vi "test first time creates file.vi"(8 "error in (no error)":errorcluster, 11 "TestCase in":refnum<class "Testing Approval Tests.lvclass">) -> (0 "error out":errorcluster, 3 "TestCase out":refnum<class "Testing Approval Tests.lvclass">)   [LabVIEW 2020, in "Testing Approval Tests.lvclass"]
uses:
  Testing Approval Tests.lvclass
  <vilib>/addons/_JKI Toolkits/VI Tester/TestCase.llb/TestCase.lvclass
  C:/Program Files/National Instruments/LabVIEW 2020/vi.lib/addons/_JKI Toolkits/VI Tester/TestCase.llb/TestCase.lvclass
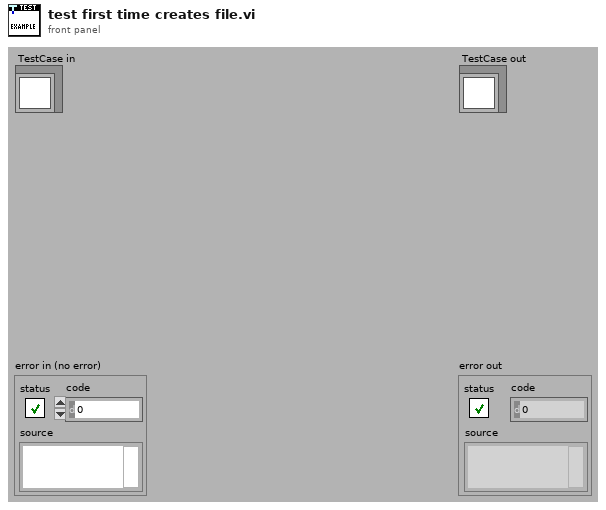
[diagram p1: front panel]
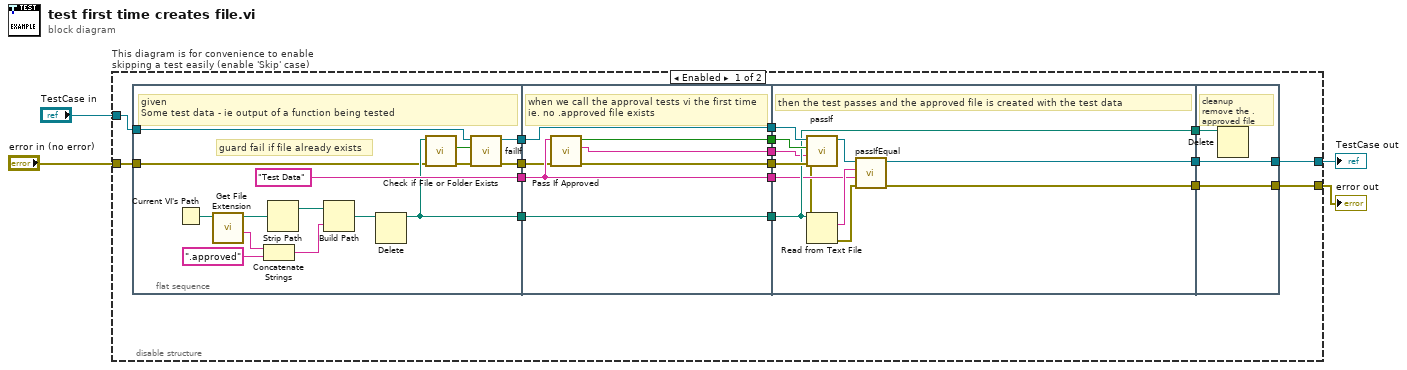
[diagram p0: block diagram]
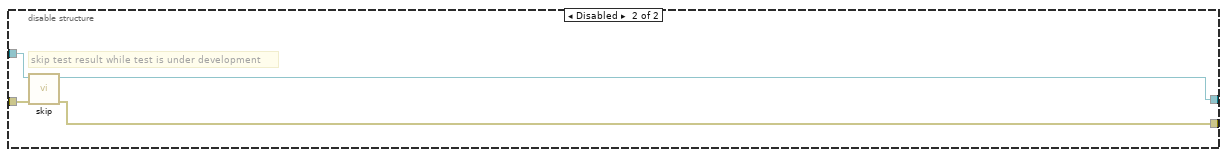
[diagram p2: hidden frame]
diagram:
  n1 = disable-structure "This diagram is for convenience to enable skipping a test easily (enable 'Skip' case)" shown="Enabled" {
    disable-tunnel: "TestCase in" -> [w19 w62]
    disable-tunnel: [w17 w60] -> w1
    disable-tunnel: [w13 w61] -> w3
    disable-tunnel: "error in (no error)" -> [w16 w59]
    frame Enabled {
      n2 = flat-sequence {
        tunnel: [w26] -> w20
        tunnel: w19 -> [w27]
        tunnel: w16 -> [w24]
        tunnel: [w28] -> w15
        tunnel: ["Test Data"] -> w10
        tunnel: [w25] -> w8
        tunnel: [w43] -> w21
        tunnel: w20 -> [w43]
        tunnel: w15 -> [w39]
        tunnel: [w38] -> w14
        tunnel: [w42] -> w11
        tunnel: w10 -> [w40]
        tunnel: [w41] -> w9
        tunnel: w8 -> [w41]
        tunnel: [w40] -> w6
        tunnel: [w37] -> w5
        tunnel: w21 -> [w55]
        tunnel: [w49] -> w18
        tunnel: w14 -> [w53]
        tunnel: [w51] -> w12
        tunnel: w11 -> [w54]
        tunnel: w9 -> [w52]
        tunnel: [w52] -> w7
        tunnel: w6 -> [w47]
        tunnel: w5 -> [w45]
        tunnel: w18 -> [w58]
        tunnel: [w58] -> w17
        tunnel: [w57] -> w13
        tunnel: w12 -> [w57]
        tunnel: w7 -> [w56]
        frame #0 {
          # "guard fail if file already exists"
          # "given\nSome test data - ie output of a function being tested"
          n3 = Current VI's Path() -> (path=w35:path)
          n4 = call <vilib>:"Get File Extension.vi"("file"=w35) -> ("filename without extension"=w32:string, "dup file"=w34:path)  [unwired: 6 in, 3 out]
          n5 = Concatenate Strings(w32, ".approved" ("string")) -> (w30:string)
          n6 = Strip Path(path=w34) -> (stripped path=w33:path)  [unwired: 1 out]
          n7 = Build Path(base path=w33, name or relative path=w30) -> (appended path=w29:path)
          n8 = Delete(path (use dialog)=w29) -> (deleted path=w25:path)  [unwired: 4 in, 2 out]
          n9 = call <vilib>:"Check if File or Folder Exists.vi"("error in (no error)"=w24, "path"=w25) -> ("error out"=w23:errorcluster, "file or folder exists?"=w22:bool)  [unwired: 7 in, 1 out]
          n10 = call-dynamic "failIf.vi"("error in (no error)"=w23, "fail"=w22, "TestCase in"=w27) -> ("error out"=w28:errorcluster, "TestCase out"=w26:refnum<class "Testing Approval Tests.lvclass">)  [unwired: 7 in]
        }
        frame #1 {
          # "when we call the approval tests vi the first time\nie. no .approved file exists"
          n11 = call "Pass If Approved.vi"("error in (no error)"=w39, "Test Data"=w40) -> ("error out"=w38:errorcluster, "Failure Message"=w37:string, "Passed?"=w42:bool)  [unwired: 7 in]
        }
        frame #2 {
          # "then the test passes and the approved file is created with the test data"
          n12 = call-dynamic "passIf.vi"("error in (no error)"=w53, "message (\"\")"=w45, "pass"=w54, "TestCase in"=w55) -> ("error out"=w44:errorcluster, "TestCase out"=w50:refnum<class "Testing Approval Tests.lvclass">)  [unwired: 6 in]
          n13 = Read from Text File(file (use dialog)=w52, error in=w44) -> (text=w48:string, error out=w46:errorcluster)  [unwired: 2 in, 2 out]
          n14 = call-dynamic "passIfEqual.vi"("error in (no error)"=w46, "y"=w47, "x"=w48, "TestCase in"=w50) -> ("error out"=w51:errorcluster, "TestCase out"=w49:refnum<class "Testing Approval Tests.lvclass">)  [unwired: 6 in]
        }
        frame #3 {
          # "cleanup \nremove the .approved file"
          n15 = Delete(path (use dialog)=w56) -> ()  [unwired: 4 in, 3 out]
        }
      }
    }
    frame Disabled {
      # "skip test result while test is under development"
      n16 = call <vilib>:"skip.vi"("error in (no error)"=w59, "TestCase in"=w62) -> ("error out"=w61:errorcluster, "TestCase out"=w60:refnum<class "Testing Approval Tests.lvclass">)  [unwired: 8 in]
    }
  }
  "error out" <- w3
  "TestCase out" <- w1
